vi "Host.vi"() -> ()   [LabVIEW 2018]
uses:
  <instrlib>/niDCPower/nidcpower.llb/niDCPower Measurement Type.ctl
panel:
  in  "PWE, мс":u32=1
  in  "5":refnum<k15>="PXI1Slot9_2" caption="instrument handle"
  in  "PWE_CMOS":bool
  in  "PWE_CCD":bool
  in  "4.1_selcur":dbl=0.02 caption="current limit" format="%_6p"
  out "4.1":i32
  out "4.1":bool
  in  "4.0_selcur":dbl=0.35 caption="current limit" format="%_6p"
  out "4.0":i32
  out "4.0":bool
  in  "4.1, V":dbl=15.0 caption="voltage level" format="%_6p"
  in  "4.1_cl, A":dbl=0.1 caption="current limit" format="%_6p"
  out "4.1_cur, A":dbl caption="measurement" format="%_6g"
  out "4.1 Chart":dbl(graph)=-0.002263378745703706 caption="Waveform Chart 5"
  in  "4.0, V":dbl=4.0 caption="voltage level" format="%_6p"
  in  "4.0_cl, A":dbl=0.4 caption="current limit" format="%_6p"
  out "4.0_cur, A":dbl caption="measurement" format="%_6g"
  out "4.0 Chart":dbl(graph)=0.0390164550609864 caption="Waveform Chart 5"
  in  "3.2_selcur":dbl=0.075 caption="current limit" format="%_6p"
  out "3.2":i32
  out "3.2":bool
  in  "3.2, V":dbl=-5.0 caption="voltage level" format="%_6p"
  in  "3.2_cl, A":dbl=0.1 caption="current limit" format="%_6p"
  out "3.2_cur, A":dbl caption="measurement" format="%_6g"
  out "3.2 Chart":dbl(graph)=-0.007994936055928669 caption="Waveform Chart 5"
  in  "2.2_selcur":dbl=0.08 caption="current limit" format="%_6p"
  out "2.2":i32
  out "2.2":bool
  out "2.2_cur, A":dbl caption="measurement" format="%_6g"
  out "2.2 Chart":dbl(graph)=-0.000235222149982668
  in  "2.2, V":dbl=-5.0 caption="voltage level" format="%_6p"
  in  "2.2_cl, A":dbl=0.1 caption="current limit" format="%_6p"
  in  "1.2_selcur":dbl=0.08 caption="current limit" format="%_6p"
  out "1.2":i32
  out "1.2":bool
  in  "1.2_cl, A":dbl=0.1 caption="current limit" format="%_6p"
  out "1.2_cur, A":dbl caption="measurement" format="%_6g"
  in  "1.2, V":dbl=-9.0 caption="voltage level" format="%_6p"
  out "1.2 Chart":dbl(graph)=-0.0025072983641264367
  out "SEL_CMOS":bool
  in  "SIM_SEL_CMOS":bool
  in  "Питание КМОП":bool
  in  "3.1_selcur":dbl=0.05 caption="current limit" format="%_6p"
  out "3.1":i32
  out "3.1":bool
  in  "3.0_selcur":dbl=15.0 caption="current limit" format="%_6p"
  out "3.0":i32
  out "3.0":bool
  in  "5.1, V":dbl=5.0 caption="voltage level" format="%_6p"
  in  "5.1_cl, A":dbl=0.1 caption="current limit" format="%_6p"
  in  "5.0, V":dbl=5.0 caption="voltage level" format="%_6p"
  in  "5.0_cl, A":dbl=0.1 caption="current limit" format="%_6p"
  in  "3.1, V":dbl=16.5 caption="voltage level" format="%_6p"
  in  "3.1_cl, A":dbl=0.1 caption="current limit" format="%_6p"
  out "3.1_cur, A":dbl caption="measurement" format="%_6g"
  out "3.1 Chart":dbl(graph)=-0.007994936055928669 caption="Waveform Chart 5"
  in  "4":refnum<k15>="PXI1Slot8_3" caption="instrument handle"
  in  "Период опроса, мс":u32=1
  out "3.0_cur, A":dbl caption="measurement" format="%_6g"
  out "3.0 Chart":dbl(graph)=0.03234747481509968 caption="Waveform Chart 5"
  in  "3.0, V":dbl=5.0 caption="voltage level" format="%_6p"
  in  "3.0_cl, A":dbl=0.02 caption="current limit" format="%_6p"
  in  "3":refnum<k15>="PXI1Slot7" caption="instrument handle"
  in  "2.1_selcur":dbl=0.05 caption="current limit" format="%_6p"
  out "2.1":i32
  out "2.1":bool
  out "2.1_cur, A":dbl caption="measurement" format="%_6g"
  out "2.1 Chart":dbl(graph)=-0.000235222149982668
  in  "2.1, V":dbl=5.0 caption="voltage level" format="%_6p"
  in  "2.1_cl, A":dbl=0.1 caption="current limit" format="%_6p"
  in  "Стоп":bool
  in  "Питание CCD":bool
  in  "SIM_SEL_CCD":bool
  out "SEL_CCD":bool
  in  "1.0_selcur":dbl=0.5 caption="current limit" format="%_6p"
  in  "1.1_selcur":dbl=0.12 caption="current limit" format="%_6p"
  in  "2.0_sel":dbl=0.25 caption="current limit" format="%_6p"
  out "1.0":i32
  out "1.0":bool
  out "1.1":i32
  out "1.1":bool
  out "2.0":i32
  out "2.0":bool
  in  "1.0, V":dbl=1.8 caption="voltage level" format="%_6p"
  in  "1.0_cl, A":dbl=0.6 caption="current limit" format="%_6p"
  in  "1.1_cl, A":dbl=0.15 caption="current limit" format="%_6p"
  out "1.0_cur, A":dbl caption="measurement" format="%_6g"
  out "1.1_cur, A":dbl caption="measurement" format="%_6g"
  in  "1.1, V":dbl=1.8 caption="voltage level" format="%_6p"
  in  "2.0, V":dbl=5.0 caption="voltage level" format="%_6p"
  in  "2.0_cl, A":dbl=0.3 caption="current limit" format="%_6p"
  out "2.0_cur, A":dbl caption="measurement" format="%_6g"
  out "1.1 Chart":dbl(graph)=-0.0025072983641264367
  out "2.0 Chart":dbl(graph)=-0.0403673797130392
  out "1.0 Chart":dbl(graph)=0.17110122624002952 caption="Waveform Chart 5"
  in  "1":refnum<k15>="PXI1Slot5_2" caption="instrument handle"
  in  "2":refnum<k15>="PXI1Slot6" caption="instrument handle"
  in  "SEL":path=path "C:/VPL/LabView/Lepton/SEL"
  out "Номер образца КМОП_ПЗС":string="0"
  # "4.0 = 4,0 CMOS 310 мА\n4.1 = SU 32 В CCD 2 мА"
  # "1.0 = 1,8_1 CMOS 400 мА\n1.1 = 1,8_2 CMOS 35-100 мА\n1.2 = - 9 CCD 60 мА"
  # "2.0 = 5,0_1 CMOS 210 мА\n2.1 = 5,0_2 CMOS 32 мА\n2.2 = - 5_1 CCD 65 мА"
  # "3.0 = 5 CCD 8 мА\n3.1 = 16,5 CCD 35 мА\n3.2 = - 5_2 CCD 60 мА"
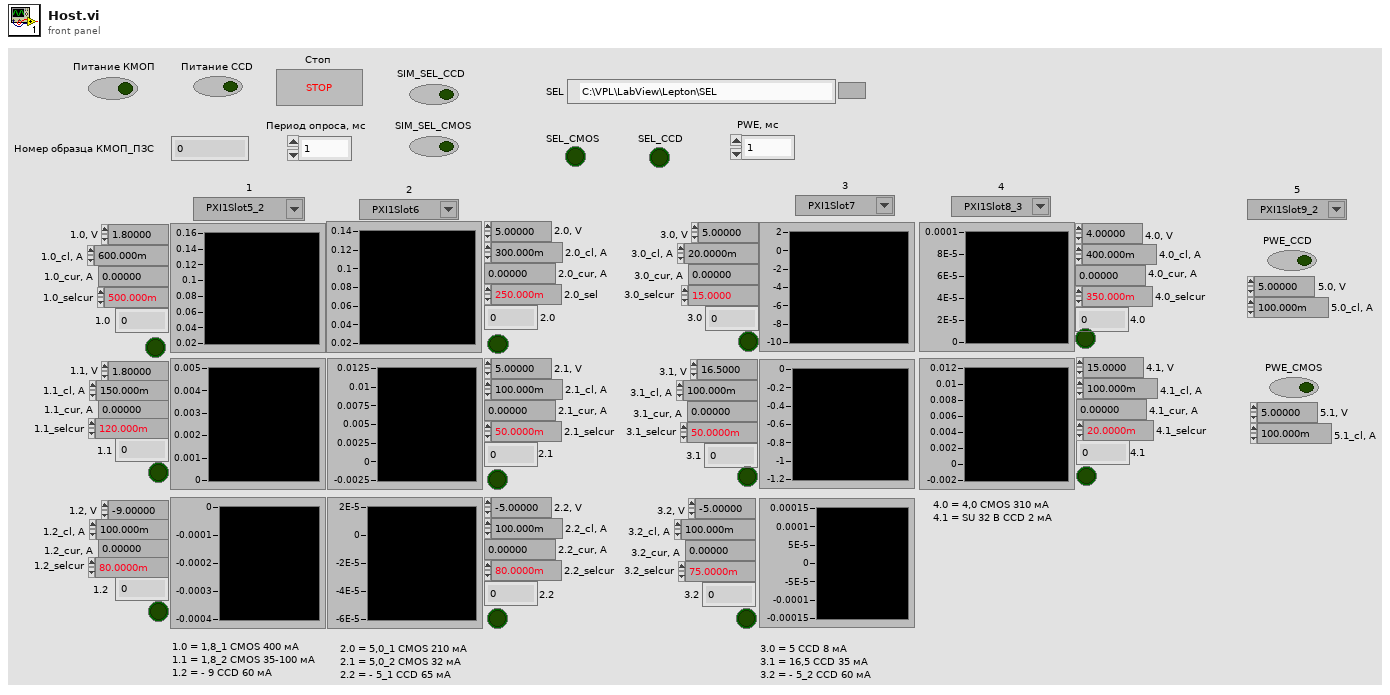
[diagram p1: front panel]
types:
  T1 = enum16{"open", "replace", "create", "open or create", "replace or create", "replace or create with confirmation"}
  T2 = typedef "niDCPower Measurement Type.ctl" = i32
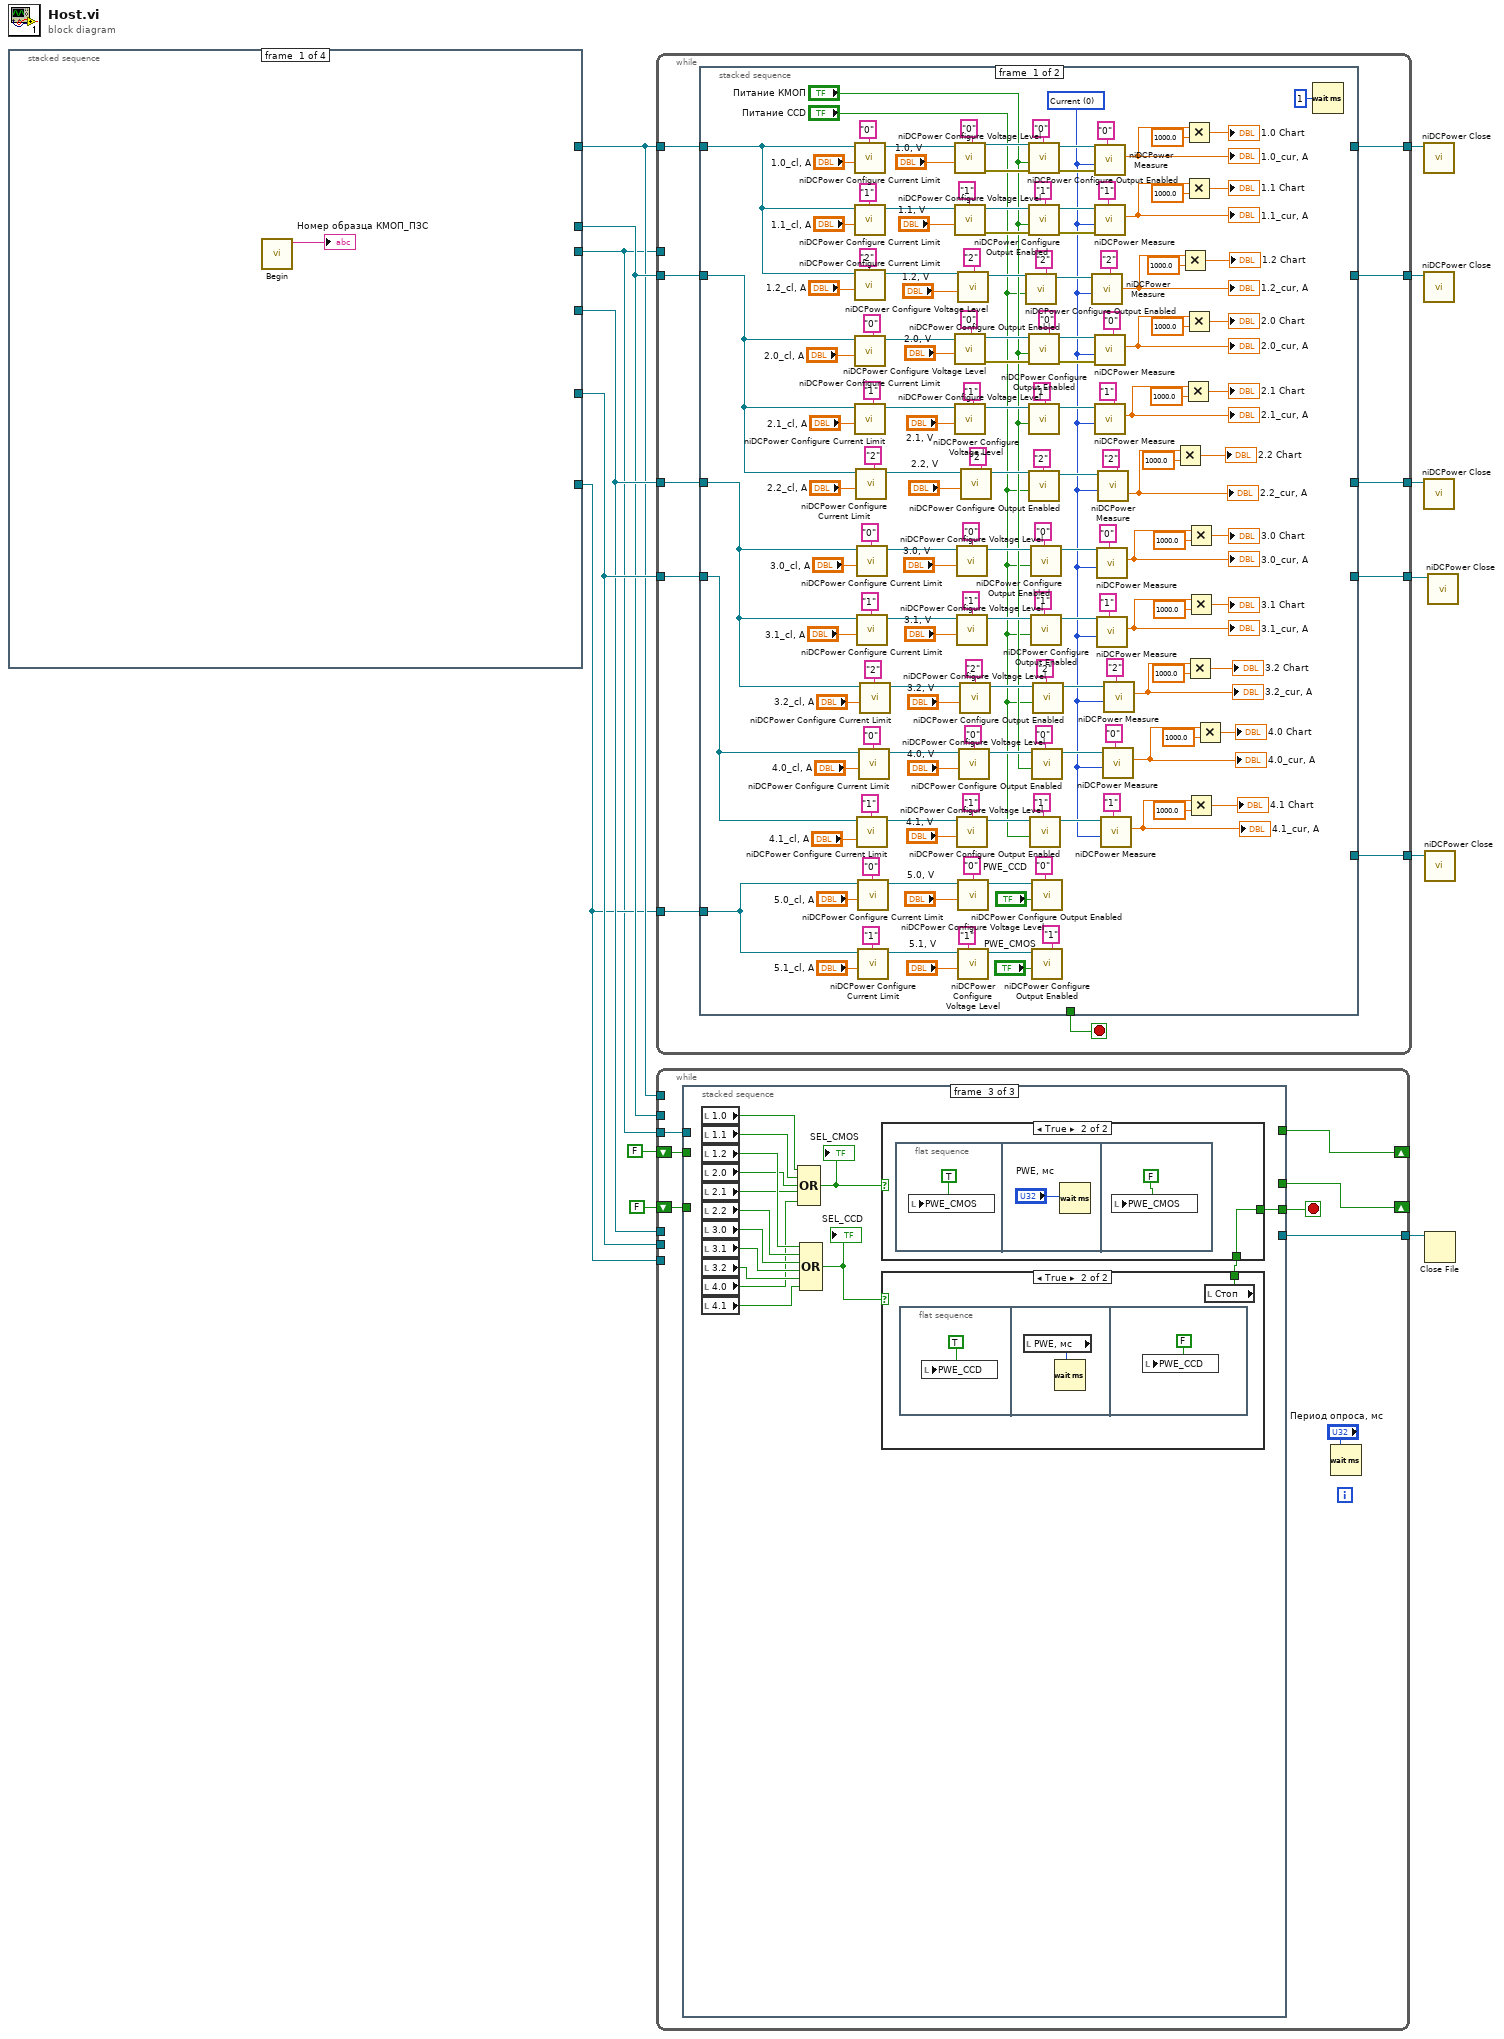
[diagram p0: block diagram]
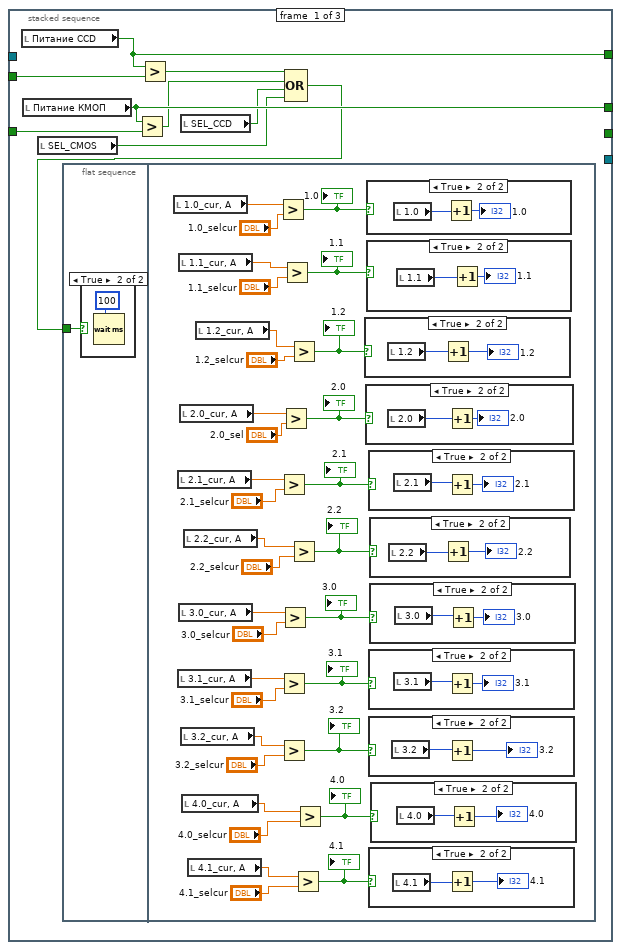
[diagram p2: hidden frame]
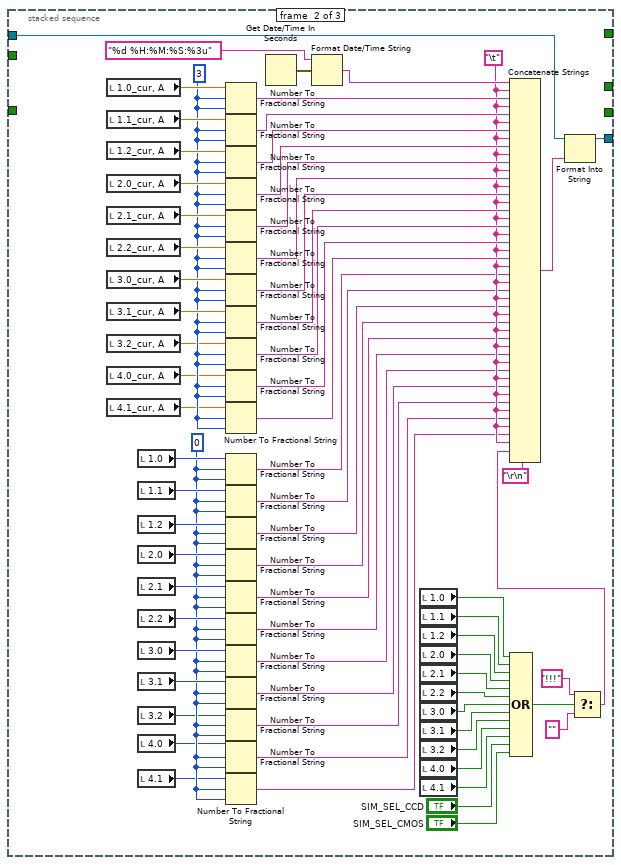
[diagram p15: hidden frame]
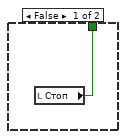
[diagram p16: hidden frame]
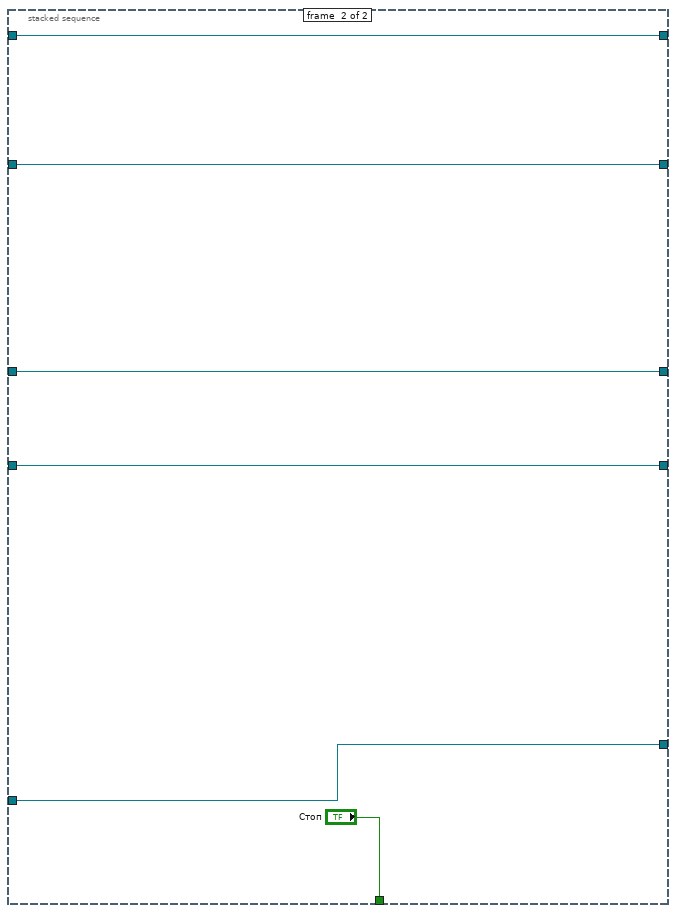
[diagram p18: hidden frame]
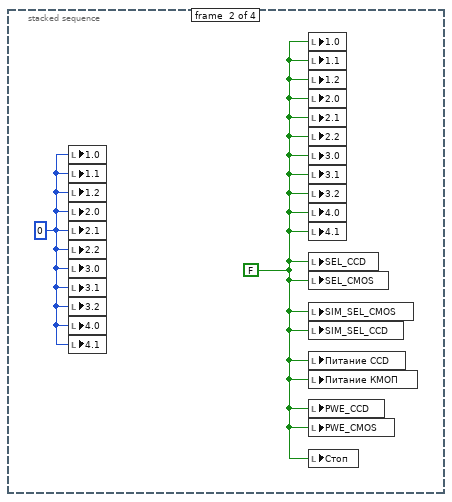
[diagram p19: hidden frame]
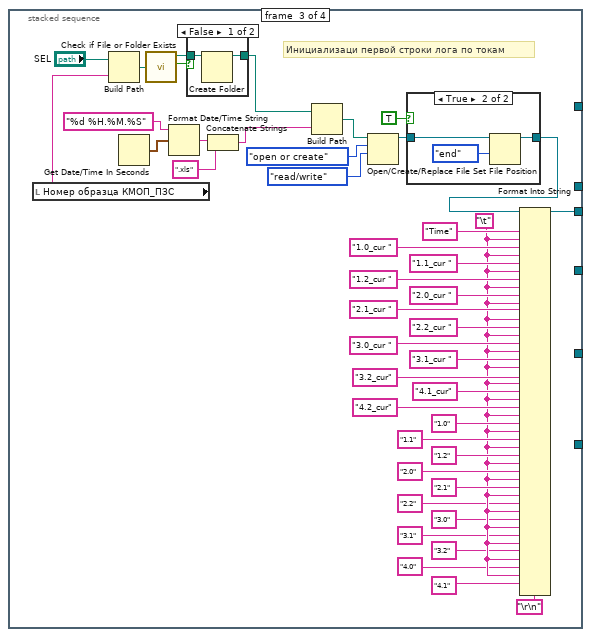
[diagram p20: hidden frame]
diagram:
  n1 = stacked-sequence {
    tunnel: [_ _ _ w87] -> w10
    tunnel: [_ _ _ w86] -> w9
    tunnel: [_ _ w44 _] -> w1
    tunnel: [_ _ _ w80] -> w11
    tunnel: [_ _ _ w74] -> w12
    tunnel: [_ _ _ w68] -> w3
    frame #0 {
      n2 = call "Begin.vi"() -> ("Номер образца 2"=→"Номер образца КМОП_ПЗС":string)  [unwired: 11 in]
    }
    frame #1 {
      w17 = 0
      w16 = FALSE
      n3 = local write "1.0"(w17) -> ()
      n4 = local write "1.1"(w17) -> ()
      n5 = local write "1.2"(w17) -> ()
      n6 = local write "2.0"(w17) -> ()
      n7 = local write "2.1"(w17) -> ()
      n8 = local write "2.2"(w17) -> ()
      n9 = local write "3.0"(w17) -> ()
      n10 = local write "3.1"(w17) -> ()
      n11 = local write "3.2"(w17) -> ()
      n12 = local write "4.0"(w17) -> ()
      n13 = local write "4.1"(w17) -> ()
      n14 = local write "1.0"(w16) -> ()
      n15 = local write "1.1"(w16) -> ()
      n16 = local write "1.2"(w16) -> ()
      n17 = local write "2.0"(w16) -> ()
      n18 = local write "2.1"(w16) -> ()
      n19 = local write "2.2"(w16) -> ()
      n20 = local write "3.0"(w16) -> ()
      n21 = local write "3.1"(w16) -> ()
      n22 = local write "3.2"(w16) -> ()
      n23 = local write "4.0"(w16) -> ()
      n24 = local write "4.1"(w16) -> ()
      n25 = local write "SEL_CCD"(w16) -> ()
      n26 = local write "SEL_CMOS"(w16) -> ()
      n27 = local write "SIM_SEL_CMOS"(w16) -> ()
      n28 = local write "SIM_SEL_CCD"(w16) -> ()
      n29 = local write "Питание CCD"(w16) -> ()
      n30 = local write "Питание КМОП"(w16) -> ()
      n31 = local write "PWE_CCD"(w16) -> ()
      n32 = local write "PWE_CMOS"(w16) -> ()
      n33 = local write "Стоп"(w16) -> ()
    }
    frame #2 {
      w25 = "\t"
      # "Инициализаци первой строки лога по токам"
      n34 = local read "Номер образца КМОП_ПЗС"() -> (w56:string)
      n35 = Build Path(base path="SEL", name or relative path=w56) -> (appended path=w58:path)
      n36 = Get Date/Time In Seconds() -> (seconds since 1Jan1904=w51:timestamp)
      n37 = call <vilib>:"Check if File or Folder Exists.vi"("path"=w58) -> ("file or folder exists?"=w59:bool, "dup path"=w60:path)  [unwired: 8 in, 1 out]
      n38 = Format Date/Time String(time format string (%c)="%d %H.%M.%S", seconds (now)=w51) -> (date/time string=w48:string)  [unwired: 1 in]
      n39 = case shown="False" w59 {
        tunnel: w60 -> [w66 w67]
        tunnel: [w65 w67] -> w43
        frame False {
          n40 = Create Folder(path (use dialog)=w66) -> (created path=w65:path)  [unwired: 2 in, 2 out]
        }
        frame True {
        }
      }
      n41 = Concatenate Strings(w48, ".xls" ("string")) -> (w46:string)
      n42 = Build Path(base path=w43, name or relative path=w46) -> (appended path=w49:path)
      n43 = Open/Create/Replace File(file path (use dialog)=w49, operation (0:open)=T1."open or create", access (0:read/write)=enum16{"read/write", "read-only", "write-only"}."read/write") -> (refnum out=w52:refnum<file>)  [unwired: 3 in, 2 out]
      n44 = case shown="True" TRUE {
        tunnel: w52 -> [w61 w64]
        tunnel: [w61 w62] -> w45
        frame False {
        }
        frame True {
          n45 = Set File Position(refnum=w64, from (0:start)=enum16{"start", "end", "current"}."end") -> (refnum out=w62:refnum<file>)  [unwired: 2 in, 1 out]
        }
      }
      n46 = Format Into String(initial string=w45, "Time" ("input 1"), w25, "1.0_cur " ("input 1"), w25, "1.1_cur " ("input 1"), w25, "1.2_cur " ("input 1"), w25, "2.0_cur " ("input 1"), w25, "2.1_cur " ("input 1"), w25, "2.2_cur " ("input 1"), w25, "3.0_cur " ("input 1"), w25, "3.1_cur " ("input 1"), w25, "3.2_cur" ("input 1"), w25, "4.1_cur" ("input 1"), w25, "4.2_cur" ("input 1"), w25, "1.0" ("input 1"), w25, "1.1" ("input 1"), w25, "1.2" ("input 1"), w25, "2.0" ("input 1"), w25, "2.1" ("input 1"), w25, "2.2" ("input 1"), w25, "3.0" ("input 1"), w25, "3.1" ("input 1"), w25, "3.2" ("input 1"), w25, "4.0" ("input 1"), w25, "4.1" ("input 1"), "\r\n") -> (resulting string=w44:refnum<file>)  [unwired: 2 in, 1 out]
    }
    frame #3 {
      n47 = call <instrlib>:"niDCPower Initialize.vi"("resource name"="5") -> ("error out"=w71:errorcluster, "instrument handle out"=w70:refnum<k15>)  [unwired: 3 in, 6 out]
      n48 = call <instrlib>:"niDCPower Initialize.vi"("resource name"="3") -> ("error out"=w83:errorcluster, "instrument handle out"=w82:refnum<k15>)  [unwired: 3 in, 6 out]
      n49 = call <instrlib>:"niDCPower Initialize.vi"("resource name"="1") -> ("error out"=w94:errorcluster, "instrument handle out"=w96:refnum<k15>)  [unwired: 3 in, 6 out]
      n50 = call <instrlib>:"niDCPower Initialize.vi"("resource name"="2") -> ("error out"=w95:errorcluster, "instrument handle out"=w97:refnum<k15>)  [unwired: 3 in, 6 out]
      n51 = call <instrlib>:"niDCPower Initialize.vi"("resource name"="4") -> ("error out"=w77:errorcluster, "instrument handle out"=w78:refnum<k15>)  [unwired: 3 in, 6 out]
      n52 = call <instrlib>:"niDCPower Configure Voltage Level.vi"("error in (no error)"=w71, "voltage level"=0.0, "channel name"="0,1", "instrument handle"=w70) -> ("instrument handle out"=w68:refnum<k15>)  [unwired: 6 in, 1 out]
      n53 = call <instrlib>:"niDCPower Configure Voltage Level.vi"("error in (no error)"=w94, "voltage level"=0.0, "channel name"="0,1,2", "instrument handle"=w96) -> ("instrument handle out"=w86:refnum<k15>)  [unwired: 6 in, 1 out]
      n54 = call <instrlib>:"niDCPower Configure Voltage Level.vi"("error in (no error)"=w95, "voltage level"=0.0, "channel name"="0,1,2", "instrument handle"=w97) -> ("instrument handle out"=w87:refnum<k15>)  [unwired: 6 in, 1 out]
      n55 = call <instrlib>:"niDCPower Configure Voltage Level.vi"("error in (no error)"=w83, "voltage level"=0.0, "channel name"="0,1,2", "instrument handle"=w82) -> ("instrument handle out"=w80:refnum<k15>)  [unwired: 6 in, 1 out]
      n56 = call <instrlib>:"niDCPower Configure Voltage Level.vi"("error in (no error)"=w77, "voltage level"=0.0, "channel name"="0,1", "instrument handle"=w78) -> ("instrument handle out"=w74:refnum<k15>)  [unwired: 6 in, 1 out]
    }
  }
  n57 = while {
    tunnel: w9 -> [w108]
    tunnel: w12 -> [w105]
    tunnel: w11 -> [w106]
    tunnel: w10 -> [w107]
    tunnel: [w104] -> w8
    tunnel: [w103] -> w7
    tunnel: [w102] -> w6
    tunnel: [w101] -> w5
    tunnel: [w99] -> w4
    tunnel: w3 -> [w98]
    tunnel: w1 -> [_]
    stop <- w100 stop-if-true
    n58 = stacked-sequence {
      tunnel: w105 -> [w148 w274]
      tunnel: w106 -> [w149 w275]
      tunnel: w107 -> [w150 w276]
      tunnel: w108 -> [w151 w277]
      tunnel: [_ w277] -> w104
      tunnel: [_ w276] -> w103
      tunnel: [_ w275] -> w102
      tunnel: [_ w274] -> w101
      tunnel: [_ "Стоп"] -> w100
      tunnel: [_ w272] -> w99
      tunnel: w98 -> [w179 w272]
      frame #0 {
        w132 = T2 0 items=["Current", "Voltage"] ("measurement type")
        n59 = call <instrlib>:"niDCPower Configure Current Limit.vi"("current limit"="1.0_cl, A", "channel name"="0", "instrument handle"=w151) -> ("instrument handle out"=w260:refnum<k15>)  [unwired: 7 in, 1 out]
        n60 = call <instrlib>:"niDCPower Configure Current Limit.vi"("current limit"="1.1_cl, A", "channel name"="1", "instrument handle"=w151) -> ("instrument handle out"=w261:refnum<k15>)  [unwired: 7 in, 1 out]
        n61 = call <instrlib>:"niDCPower Configure Current Limit.vi"("current limit"="1.2_cl, A", "channel name"="2", "instrument handle"=w151) -> ("instrument handle out"=w135:refnum<k15>)  [unwired: 7 in, 1 out]
        n62 = call <instrlib>:"niDCPower Configure Current Limit.vi"("current limit"="2.0_cl, A", "channel name"="0", "instrument handle"=w150) -> ("instrument handle out"=w243:refnum<k15>)  [unwired: 7 in, 1 out]
        n63 = call <instrlib>:"niDCPower Configure Current Limit.vi"("current limit"="2.1_cl, A", "channel name"="1", "instrument handle"=w150) -> ("instrument handle out"=w223:refnum<k15>)  [unwired: 7 in, 1 out]
        n64 = call <instrlib>:"niDCPower Configure Current Limit.vi"("current limit"="2.2_cl, A", "channel name"="2", "instrument handle"=w150) -> ("instrument handle out"=w138:refnum<k15>)  [unwired: 7 in, 1 out]
        n65 = call <instrlib>:"niDCPower Configure Current Limit.vi"("current limit"="3.0_cl, A", "channel name"="0", "instrument handle"=w149) -> ("instrument handle out"=w214:refnum<k15>)  [unwired: 7 in, 1 out]
        n66 = call <instrlib>:"niDCPower Configure Current Limit.vi"("current limit"="3.1_cl, A", "channel name"="1", "instrument handle"=w149) -> ("instrument handle out"=w195:refnum<k15>)  [unwired: 7 in, 1 out]
        n67 = call <instrlib>:"niDCPower Configure Current Limit.vi"("current limit"="4.1_cl, A", "channel name"="1", "instrument handle"=w148) -> ("instrument handle out"=w144:refnum<k15>)  [unwired: 7 in, 1 out]
        n68 = call <instrlib>:"niDCPower Configure Current Limit.vi"("current limit"="5.0_cl, A", "channel name"="0", "instrument handle"=w179) -> ("instrument handle out"=w191:refnum<k15>)  [unwired: 7 in, 1 out]
        n69 = call <instrlib>:"niDCPower Configure Current Limit.vi"("current limit"="5.1_cl, A", "channel name"="1", "instrument handle"=w179) -> ("instrument handle out"=w182:refnum<k15>)  [unwired: 7 in, 1 out]
        n70 = call <instrlib>:"niDCPower Configure Current Limit.vi"("current limit"="4.0_cl, A", "channel name"="0", "instrument handle"=w148) -> ("instrument handle out"=w147:refnum<k15>)  [unwired: 7 in, 1 out]
        n71 = call <instrlib>:"niDCPower Configure Current Limit.vi"("current limit"="3.2_cl, A", "channel name"="2", "instrument handle"=w149) -> ("instrument handle out"=w141:refnum<k15>)  [unwired: 7 in, 1 out]
        n72 = call <instrlib>:"niDCPower Configure Voltage Level.vi"("voltage level"="1.0, V", "channel name"="0", "instrument handle"=w260) -> ("error out"=w253:errorcluster, "instrument handle out"=w256:refnum<k15>)  [unwired: 7 in]
        n73 = call <instrlib>:"niDCPower Configure Voltage Level.vi"("voltage level"="1.1, V", "channel name"="1", "instrument handle"=w261) -> ("error out"=w254:errorcluster, "instrument handle out"=w255:refnum<k15>)  [unwired: 7 in]
        n74 = call <instrlib>:"niDCPower Configure Voltage Level.vi"("voltage level"="2.0, V", "channel name"="0", "instrument handle"=w243) -> ("error out"=w247:errorcluster, "instrument handle out"=w248:refnum<k15>)  [unwired: 7 in]
        n75 = call <instrlib>:"niDCPower Configure Voltage Level.vi"("voltage level"="2.1, V", "channel name"="1", "instrument handle"=w223) -> ("instrument handle out"=w221:refnum<k15>)  [unwired: 7 in, 1 out]
        n76 = call <instrlib>:"niDCPower Configure Voltage Level.vi"("voltage level"="3.0, V", "channel name"="0", "instrument handle"=w214) -> ("instrument handle out"=w213:refnum<k15>)  [unwired: 7 in, 1 out]
        n77 = call <instrlib>:"niDCPower Configure Voltage Level.vi"("voltage level"="3.1, V", "channel name"="1", "instrument handle"=w195) -> ("instrument handle out"=w196:refnum<k15>)  [unwired: 7 in, 1 out]
        n78 = call <instrlib>:"niDCPower Configure Voltage Level.vi"("voltage level"="4.1, V", "channel name"="1", "instrument handle"=w144) -> ("instrument handle out"=w143:refnum<k15>)  [unwired: 7 in, 1 out]
        n79 = call <instrlib>:"niDCPower Configure Voltage Level.vi"("voltage level"="1.2, V", "channel name"="2", "instrument handle"=w135) -> ("instrument handle out"=w134:refnum<k15>)  [unwired: 7 in, 1 out]
        n80 = call <instrlib>:"niDCPower Configure Voltage Level.vi"("voltage level"="5.0, V", "channel name"="0", "instrument handle"=w191) -> ("instrument handle out"=w190:refnum<k15>)  [unwired: 7 in, 1 out]
        n81 = call <instrlib>:"niDCPower Configure Voltage Level.vi"("voltage level"="5.1, V", "channel name"="1", "instrument handle"=w182) -> ("instrument handle out"=w183:refnum<k15>)  [unwired: 7 in, 1 out]
        n82 = call <instrlib>:"niDCPower Configure Voltage Level.vi"("voltage level"="4.0, V", "channel name"="0", "instrument handle"=w147) -> ("instrument handle out"=w146:refnum<k15>)  [unwired: 7 in, 1 out]
        n83 = call <instrlib>:"niDCPower Configure Voltage Level.vi"("voltage level"="3.2, V", "channel name"="2", "instrument handle"=w141) -> ("instrument handle out"=w140:refnum<k15>)  [unwired: 7 in, 1 out]
        n84 = call <instrlib>:"niDCPower Configure Voltage Level.vi"("voltage level"="2.2, V", "channel name"="2", "instrument handle"=w138) -> ("instrument handle out"=w137:refnum<k15>)  [unwired: 7 in, 1 out]
        n85 = call <instrlib>:"niDCPower Configure Output Enabled.vi"("output enabled"="Питание CCD", "channel name"="2", "instrument handle"=w134) -> ("instrument handle out"=w133:refnum<k15>)  [unwired: 7 in, 1 out]
        n86 = call <instrlib>:"niDCPower Configure Output Enabled.vi"("error in (no error)"=w253, "output enabled"="Питание КМОП", "channel name"="0", "instrument handle"=w256) -> ("error out"=w265:errorcluster, "instrument handle out"=w264:refnum<k15>)  [unwired: 6 in]
        n87 = call <instrlib>:"niDCPower Configure Output Enabled.vi"("error in (no error)"=w254, "output enabled"="Питание КМОП", "channel name"="1", "instrument handle"=w255) -> ("error out"=w266:errorcluster, "instrument handle out"=w267:refnum<k15>)  [unwired: 6 in]
        n88 = call <instrlib>:"niDCPower Configure Output Enabled.vi"("error in (no error)"=w247, "output enabled"="Питание КМОП", "channel name"="0", "instrument handle"=w248) -> ("error out"=w239:errorcluster, "instrument handle out"=w240:refnum<k15>)  [unwired: 6 in]
        n89 = call <instrlib>:"niDCPower Configure Output Enabled.vi"("output enabled"="Питание КМОП", "channel name"="1", "instrument handle"=w221) -> ("instrument handle out"=w219:refnum<k15>)  [unwired: 7 in, 1 out]
        n90 = call <instrlib>:"niDCPower Configure Output Enabled.vi"("output enabled"="Питание CCD", "channel name"="2", "instrument handle"=w137) -> ("instrument handle out"=w136:refnum<k15>)  [unwired: 7 in, 1 out]
        n91 = call <instrlib>:"niDCPower Configure Output Enabled.vi"("output enabled"="Питание CCD", "channel name"="1", "instrument handle"=w143) -> ("instrument handle out"=w142:refnum<k15>)  [unwired: 7 in, 1 out]
        n92 = call <instrlib>:"niDCPower Configure Output Enabled.vi"("output enabled"="Питание CCD", "channel name"="0", "instrument handle"=w213) -> ("instrument handle out"=w212:refnum<k15>)  [unwired: 7 in, 1 out]
        n93 = call <instrlib>:"niDCPower Configure Output Enabled.vi"("output enabled"="Питание CCD", "channel name"="1", "instrument handle"=w196) -> ("instrument handle out"=w197:refnum<k15>)  [unwired: 7 in, 1 out]
        n94 = call <instrlib>:"niDCPower Configure Output Enabled.vi"("output enabled"="Питание КМОП", "channel name"="0", "instrument handle"=w146) -> ("instrument handle out"=w145:refnum<k15>)  [unwired: 7 in, 1 out]
        n95 = call <instrlib>:"niDCPower Configure Output Enabled.vi"("output enabled"="PWE_CCD", "channel name"="0", "instrument handle"=w190) -> ()  [unwired: 7 in, 2 out]
        n96 = call <instrlib>:"niDCPower Configure Output Enabled.vi"("output enabled"="PWE_CMOS", "channel name"="1", "instrument handle"=w183) -> ()  [unwired: 7 in, 2 out]
        n97 = call <instrlib>:"niDCPower Configure Output Enabled.vi"("output enabled"="Питание CCD", "channel name"="2", "instrument handle"=w140) -> ("instrument handle out"=w139:refnum<k15>)  [unwired: 7 in, 1 out]
        n98 = call <instrlib>:"niDCPower Measure.vi"("measurement type"=w132, "channel name"="2", "instrument handle"=w133) -> ("measurement"=w109:dbl)  [unwired: 6 in, 2 out]
        "1.2_cur, A" <- w109
        n99 = call <instrlib>:"niDCPower Measure.vi"("error in (no error)"=w265, "measurement type"=w132, "channel name"="0", "instrument handle"=w264) -> ("measurement"=w232:dbl)  [unwired: 5 in, 2 out]
        "1.0_cur, A" <- w232
        n100 = call <instrlib>:"niDCPower Measure.vi"("error in (no error)"=w266, "measurement type"=w132, "channel name"="1", "instrument handle"=w267) -> ("measurement"=w235:dbl)  [unwired: 5 in, 2 out]
        "1.1_cur, A" <- w235
        n101 = call <instrlib>:"niDCPower Measure.vi"("error in (no error)"=w239, "measurement type"=w132, "channel name"="0", "instrument handle"=w240) -> ("measurement"=w233:dbl)  [unwired: 5 in, 2 out]
        "2.0_cur, A" <- w233
        n102 = call <instrlib>:"niDCPower Measure.vi"("measurement type"=w132, "channel name"="1", "instrument handle"=w219) -> ("measurement"=w217:dbl)  [unwired: 6 in, 2 out]
        "2.1_cur, A" <- w217
        n103 = call <instrlib>:"niDCPower Measure.vi"("measurement type"=w132, "channel name"="0", "instrument handle"=w212) -> ("measurement"=w211:dbl)  [unwired: 6 in, 2 out]
        "3.0_cur, A" <- w211
        n104 = call <instrlib>:"niDCPower Measure.vi"("measurement type"=w132, "channel name"="1", "instrument handle"=w197) -> ("measurement"=w198:dbl)  [unwired: 6 in, 2 out]
        "3.1_cur, A" <- w198
        n105 = call <instrlib>:"niDCPower Measure.vi"("measurement type"=w132, "channel name"="2", "instrument handle"=w136) -> ("measurement"=w111:dbl)  [unwired: 6 in, 2 out]
        "2.2_cur, A" <- w111
        n106 = call <instrlib>:"niDCPower Measure.vi"("measurement type"=w132, "channel name"="1", "instrument handle"=w142) -> ("measurement"=w117:dbl)  [unwired: 6 in, 2 out]
        "4.1_cur, A" <- w117
        n107 = call <instrlib>:"niDCPower Measure.vi"("measurement type"=w132, "channel name"="0", "instrument handle"=w145) -> ("measurement"=w116:dbl)  [unwired: 6 in, 2 out]
        "4.0_cur, A" <- w116
        n108 = call <instrlib>:"niDCPower Measure.vi"("measurement type"=w132, "channel name"="2", "instrument handle"=w139) -> ("measurement"=w114:dbl)  [unwired: 6 in, 2 out]
        "3.2_cur, A" <- w114
        n109 = Multiply(x=w111, y=1000.0) -> (x*y=→"2.2 Chart":dbl)
        n110 = Multiply(x=w109, y=1000.0) -> (x*y=→"1.2 Chart":dbl)
        n111 = Multiply(x=w217, y=1000.0) -> (x*y=→"2.1 Chart":dbl)
        n112 = Multiply(x=w232, y=1000.0) -> (x*y=→"1.0 Chart":dbl)
        n113 = Multiply(x=w235, y=1000.0) -> (x*y=→"1.1 Chart":dbl)
        n114 = Multiply(x=w233, y=1000.0) -> (x*y=→"2.0 Chart":dbl)
        n115 = Multiply(x=w114, y=1000.0) -> (x*y=→"3.2 Chart":dbl)
        n116 = Multiply(x=w211, y=1000.0) -> (x*y=→"3.0 Chart":dbl)
        n117 = Multiply(x=w198, y=1000.0) -> (x*y=→"3.1 Chart":dbl)
        n118 = Multiply(x=w117, y=1000.0) -> (x*y=→"4.1 Chart":dbl)
        n119 = Multiply(x=w116, y=1000.0) -> (x*y=→"4.0 Chart":dbl)
        n120 = Wait (ms)(milliseconds to wait=u32 1) -> ()  [unwired: 1 out]
      }
      frame #1 {
      }
    }
  }
  n121 = while {
    shift-right: [w285] -> _
    shift-left: FALSE -> [w284]
    tunnel: w1 -> [w283]
    tunnel: [w282] -> w13
    tunnel: w12 -> [_]
    tunnel: w11 -> [_]
    tunnel: w10 -> [_]
    tunnel: w9 -> [_]
    tunnel: w3 -> [_]
    shift-right: [w279] -> _
    shift-left: FALSE -> [w280]
    stop <- w278 stop-if-true
    n122 = stacked-sequence {
      tunnel: [w292 _ _] -> w285
      tunnel: w284 -> [w294 _ _]
      tunnel: w283 -> [_ w415 _]
      tunnel: [_ w413 _] -> w282
      tunnel: w280 -> [w293 _ _]
      tunnel: [w291 _ _] -> w279
      tunnel: [_ _ w426] -> w278
      frame #0 {
        n123 = local read "Питание CCD"() -> (w292:bool)
        n124 = local read "Питание КМОП"() -> (w291:bool)
        n125 = local read "SEL_CMOS"() -> (w287:bool)
        n126 = flat-sequence {
          tunnel: w286 -> [w295]
          frame #0 {
            n127 = case shown="True" w295 {
              frame False {
              }
              frame True {
                n128 = Wait (ms)(milliseconds to wait=u32 100) -> ()  [unwired: 1 out]
              }
            }
          }
          frame #1 {
            n129 = local read "1.0_cur, A"() -> (w323:dbl)
            n130 = local read "2.1_cur, A"() -> (w320:dbl)
            n131 = local read "3.1_cur, A"() -> (w314:dbl)
            n132 = local read "1.1_cur, A"() -> (w322:dbl)
            n133 = local read "3.0_cur, A"() -> (w315:dbl)
            n134 = local read "2.0_cur, A"() -> (w321:dbl)
            n135 = local read "3.2_cur, A"() -> (w299:dbl)
            n136 = local read "4.0_cur, A"() -> (w298:dbl)
            n137 = local read "2.2_cur, A"() -> (w300:dbl)
            n138 = local read "4.1_cur, A"() -> (w297:dbl)
            n139 = local read "1.2_cur, A"() -> (w301:dbl)
            n140 = Greater?(x=w323, y="1.0_selcur") -> (0:w328:bool)
            "1.0" <- w328
            n141 = Greater?(x=w320, y="2.1_selcur") -> (0:w319:bool)
            "2.1" <- w319
            n142 = Greater?(x=w314, y="3.1_selcur") -> (0:w313:bool)
            "3.1" <- w313
            n143 = Greater?(x=w299, y="3.2_selcur") -> (0:w309:bool)
            "3.2" <- w309
            n144 = Greater?(x=w315, y="3.0_selcur") -> (0:w316:bool)
            "3.0" <- w316
            n145 = Greater?(x=w321, y="2.0_sel") -> (0:w324:bool)
            "2.0" <- w324
            n146 = Greater?(x=w322, y="1.1_selcur") -> (0:w326:bool)
            "1.1" <- w326
            n147 = Greater?(x=w301, y="1.2_selcur") -> (0:w311:bool)
            "1.2" <- w311
            n148 = Greater?(x=w300, y="2.2_selcur") -> (0:w310:bool)
            "2.2" <- w310
            n149 = Greater?(x=w297, y="4.1_selcur") -> (0:w307:bool)
            "4.1" <- w307
            n150 = Greater?(x=w298, y="4.0_selcur") -> (0:w308:bool)
            "4.0" <- w308
            n151 = case shown="True" w311 {
              frame False {
              }
              frame True {
                n152 = local read "1.2"() -> (w331:i32)
                n153 = Increment(x=w331) -> (x+1=→"1.2":i32)
              }
            }
            n154 = case shown="True" w324 {
              frame False {
              }
              frame True {
                n155 = local read "2.0"() -> (w347:i32)
                n156 = Increment(x=w347) -> (x+1=→"2.0":i32)
              }
            }
            n157 = case shown="True" w328 {
              frame False {
              }
              frame True {
                n158 = local read "1.0"() -> (w351:i32)
                n159 = Increment(x=w351) -> (x+1=→"1.0":i32)
              }
            }
            n160 = case shown="True" w326 {
              frame False {
              }
              frame True {
                n161 = local read "1.1"() -> (w348:i32)
                n162 = Increment(x=w348) -> (x+1=→"1.1":i32)
              }
            }
            n163 = case shown="True" w319 {
              frame False {
              }
              frame True {
                n164 = local read "2.1"() -> (w345:i32)
                n165 = Increment(x=w345) -> (x+1=→"2.1":i32)
              }
            }
            n166 = case shown="True" w313 {
              frame False {
              }
              frame True {
                n167 = local read "3.1"() -> (w341:i32)
                n168 = Increment(x=w341) -> (x+1=→"3.1":i32)
              }
            }
            n169 = case shown="True" w309 {
              frame False {
              }
              frame True {
                n170 = local read "3.2"() -> (w338:i32)
                n171 = Increment(x=w338) -> (x+1=→"3.2":i32)
              }
            }
            n172 = case shown="True" w307 {
              frame False {
              }
              frame True {
                n173 = local read "4.1"() -> (w337:i32)
                n174 = Increment(x=w337) -> (x+1=→"4.1":i32)
              }
            }
            n175 = case shown="True" w310 {
              frame False {
              }
              frame True {
                n176 = local read "2.2"() -> (w333:i32)
                n177 = Increment(x=w333) -> (x+1=→"2.2":i32)
              }
            }
            n178 = case shown="True" w316 {
              frame False {
              }
              frame True {
                n179 = local read "3.0"() -> (w343:i32)
                n180 = Increment(x=w343) -> (x+1=→"3.0":i32)
              }
            }
            n181 = case shown="True" w308 {
              frame False {
              }
              frame True {
                n182 = local read "4.0"() -> (w335:i32)
                n183 = Increment(x=w335) -> (x+1=→"4.0":i32)
              }
            }
          }
        }
        n184 = Greater?(x=w291, y=w293) -> (0:w289:bool)
        n185 = Greater?(x=w292, y=w294) -> (0:w290:bool)
        n186 = local read "SEL_CCD"() -> (w288:bool)
        n187 = Compound Arithmetic op=OR(w290, w289, w288, w287) -> (w286:bool)
      }
      frame #1 {
        w385 = i16 0 ("width (-)")
        w398 = i16 3 ("width (-)")
        w381 = "\t"
        n188 = local read "1.0_cur, A"() -> (w408:dbl)
        n189 = local read "1.1_cur, A"() -> (w407:dbl)
        n190 = local read "1.2_cur, A"() -> (w404:dbl)
        n191 = local read "2.0_cur, A"() -> (w403:dbl)
        n192 = local read "2.1_cur, A"() -> (w402:dbl)
        n193 = local read "2.2_cur, A"() -> (w401:dbl)
        n194 = local read "3.0_cur, A"() -> (w400:dbl)
        n195 = local read "3.1_cur, A"() -> (w399:dbl)
        n196 = local read "3.2_cur, A"() -> (w395:dbl)
        n197 = local read "4.0_cur, A"() -> (w396:dbl)
        n198 = local read "4.1_cur, A"() -> (w397:dbl)
        n199 = local read "1.0"() -> (w406:i32)
        n200 = local read "1.1"() -> (w405:i32)
        n201 = local read "1.2"() -> (w391:i32)
        n202 = local read "2.0"() -> (w390:i32)
        n203 = local read "2.1"() -> (w389:i32)
        n204 = local read "2.2"() -> (w388:i32)
        n205 = local read "3.0"() -> (w387:i32)
        n206 = local read "3.1"() -> (w386:i32)
        n207 = local read "3.2"() -> (w384:i32)
        n208 = local read "4.0"() -> (w383:i32)
        n209 = local read "4.1"() -> (w382:i32)
        n210 = Number To Fractional String(number=w408, width (-)=w398, precision (6)=w398) -> (F-format string=w418:string)  [unwired: 1 in]
        n211 = Number To Fractional String(number=w407, width (-)=w398, precision (6)=w398) -> (F-format string=w417:string)  [unwired: 1 in]
        n212 = Number To Fractional String(number=w404, width (-)=w398, precision (6)=w398) -> (F-format string=w416:string)  [unwired: 1 in]
        n213 = Number To Fractional String(number=w403, width (-)=w398, precision (6)=w398) -> (F-format string=w414:string)  [unwired: 1 in]
        n214 = Number To Fractional String(number=w402, width (-)=w398, precision (6)=w398) -> (F-format string=w412:string)  [unwired: 1 in]
        n215 = Number To Fractional String(number=w401, width (-)=w398, precision (6)=w398) -> (F-format string=w411:string)  [unwired: 1 in]
        n216 = Number To Fractional String(number=w400, width (-)=w398, precision (6)=w398) -> (F-format string=w410:string)  [unwired: 1 in]
        n217 = Number To Fractional String(number=w399, width (-)=w398, precision (6)=w398) -> (F-format string=w409:string)  [unwired: 1 in]
        n218 = Number To Fractional String(number=w395, width (-)=w398, precision (6)=w398) -> (F-format string=w394:string)  [unwired: 1 in]
        n219 = Number To Fractional String(number=w396, width (-)=w398, precision (6)=w398) -> (F-format string=w393:string)  [unwired: 1 in]
        n220 = Number To Fractional String(number=w397, width (-)=w398, precision (6)=w398) -> (F-format string=w392:string)  [unwired: 1 in]
        n221 = Number To Fractional String(number=w406, width (-)=w385, precision (6)=w385) -> (F-format string=w380:string)  [unwired: 1 in]
        n222 = Number To Fractional String(number=w405, width (-)=w385, precision (6)=w385) -> (F-format string=w379:string)  [unwired: 1 in]
        n223 = Number To Fractional String(number=w391, width (-)=w385, precision (6)=w385) -> (F-format string=w378:string)  [unwired: 1 in]
        n224 = Number To Fractional String(number=w390, width (-)=w385, precision (6)=w385) -> (F-format string=w377:string)  [unwired: 1 in]
        n225 = Number To Fractional String(number=w389, width (-)=w385, precision (6)=w385) -> (F-format string=w376:string)  [unwired: 1 in]
        n226 = Number To Fractional String(number=w388, width (-)=w385, precision (6)=w385) -> (F-format string=w375:string)  [unwired: 1 in]
        n227 = Number To Fractional String(number=w387, width (-)=w385, precision (6)=w385) -> (F-format string=w374:string)  [unwired: 1 in]
        n228 = Number To Fractional String(number=w386, width (-)=w385, precision (6)=w385) -> (F-format string=w373:string)  [unwired: 1 in]
        n229 = Number To Fractional String(number=w384, width (-)=w385, precision (6)=w385) -> (F-format string=w372:string)  [unwired: 1 in]
        n230 = Number To Fractional String(number=w383, width (-)=w385, precision (6)=w385) -> (F-format string=w371:string)  [unwired: 1 in]
        n231 = Number To Fractional String(number=w382, width (-)=w385, precision (6)=w385) -> (F-format string=w370:string)  [unwired: 1 in]
        n232 = Get Date/Time In Seconds() -> (seconds since 1Jan1904=w422:timestamp)
        n233 = Format Date/Time String(time format string (%c)="%d %H:%M:%S:%3u", seconds (now)=w422) -> (date/time string=w419:string)  [unwired: 1 in]
        n234 = local read "1.0"() -> (w368:bool)
        n235 = local read "1.1"() -> (w367:bool)
        n236 = local read "1.2"() -> (w366:bool)
        n237 = local read "2.0"() -> (w365:bool)
        n238 = local read "2.1"() -> (w364:bool)
        n239 = local read "2.2"() -> (w363:bool)
        n240 = local read "3.0"() -> (w362:bool)
        n241 = local read "3.1"() -> (w361:bool)
        n242 = local read "3.2"() -> (w360:bool)
        n243 = local read "4.0"() -> (w359:bool)
        n244 = local read "4.1"() -> (w358:bool)
        n245 = Compound Arithmetic op=OR(w368, w367, w366, w365, w364, w363, w362, w361, w360, w359, w358, "SIM_SEL_CCD", "SIM_SEL_CMOS") -> (w369:bool)
        n246 = Select(t="!!!", s=w369, f="") -> (s? t:f=w353:string)
        n247 = Concatenate Strings(w419, w381, w418, w381, w417, w381, w416, w381, w414, w381, w412, w381, w411, w381, w410, w381, w409, w381, w394, w381, w393, w381, w392, w381, w380, w381, w379, w381, w378, w381, w377, w381, w376, w381, w375, w381, w374, w381, w373, w381, w372, w381, w371, w381, w370, w381, w353, "\r\n") -> (w421:string)
        n248 = Format Into String(initial string=w415, w421) -> (resulting string=w413:refnum<file>)  [unwired: 2 in, 1 out]
      }
      frame #2 {
        n249 = local read "1.0"() -> (w437:bool)
        n250 = local read "1.1"() -> (w436:bool)
        n251 = local read "1.2"() -> (w435:bool)
        n252 = local read "2.0"() -> (w434:bool)
        n253 = local read "2.1"() -> (w433:bool)
        n254 = local read "2.2"() -> (w432:bool)
        n255 = local read "3.0"() -> (w431:bool)
        n256 = local read "3.1"() -> (w430:bool)
        n257 = local read "3.2"() -> (w429:bool)
        n258 = local read "4.0"() -> (w428:bool)
        n259 = local read "4.1"() -> (w427:bool)
        n260 = Compound Arithmetic op=OR(w437, w436, w434, w433, w428) -> (w424:bool)
        "SEL_CMOS" <- w424
        n261 = Compound Arithmetic op=OR(w435, w432, w431, w430, w429, w427) -> (w423:bool)
        "SEL_CCD" <- w423
        n262 = case shown="True" w423 {
          tunnel: [w438 w439] -> w425
          frame False {
            n263 = local read "Стоп"() -> (w438:bool)
          }
          frame True {
            n264 = flat-sequence {
              frame #0 {
                n265 = local write "PWE_CCD"(TRUE) -> ()
              }
              frame #1 {
                n266 = local read "PWE, мс"() -> (w441:u32)
                n267 = Wait (ms)(milliseconds to wait=w441) -> ()  [unwired: 1 out]
              }
              frame #2 {
                n268 = local write "PWE_CCD"(FALSE) -> ()
              }
            }
            n269 = local read "Стоп"() -> (w439:bool)
          }
        }
        n270 = case shown="True" w424 {
          tunnel: [w443 w444] -> w426
          tunnel: w425 -> [w443 w444]
          frame False {
          }
          frame True {
            n271 = flat-sequence {
              frame #0 {
                n272 = local write "PWE_CMOS"(TRUE) -> ()
              }
              frame #1 {
                n273 = Wait (ms)(milliseconds to wait="PWE, мс") -> ()  [unwired: 1 out]
              }
              frame #2 {
                n274 = local write "PWE_CMOS"(FALSE) -> ()
              }
            }
          }
        }
      }
    }
    n275 = Wait (ms)(milliseconds to wait="Период опроса, мс") -> ()  [unwired: 1 out]
  }
  n276 = call <instrlib>:"niDCPower Close.vi"("instrument handle"=w8) -> ()  [unwired: 10 in, 1 out]
  n277 = call <instrlib>:"niDCPower Close.vi"("instrument handle"=w7) -> ()  [unwired: 10 in, 1 out]
  n278 = call <instrlib>:"niDCPower Close.vi"("instrument handle"=w6) -> ()  [unwired: 10 in, 1 out]
  n279 = call <instrlib>:"niDCPower Close.vi"("instrument handle"=w4) -> ()  [unwired: 10 in, 1 out]
  n280 = Close File(refnum=w13) -> ()  [unwired: 1 in, 2 out]
  n281 = call <instrlib>:"niDCPower Close.vi"("instrument handle"=w5) -> ()  [unwired: 10 in, 1 out]
